vi "Write FPGA Setup Params to File.vi"(8 "error in (no error)":errorcluster, 11 "Path":path) -> (0 "error out":errorcluster)   [LabVIEW 2015, in "Tool Cfg.lvlib"]
uses:
  Tool Cfg.lvlib
  <vilib>/Utility/xml.llb/Write to XML File(array).vi
  Tool Module/Tool Module.lvlib
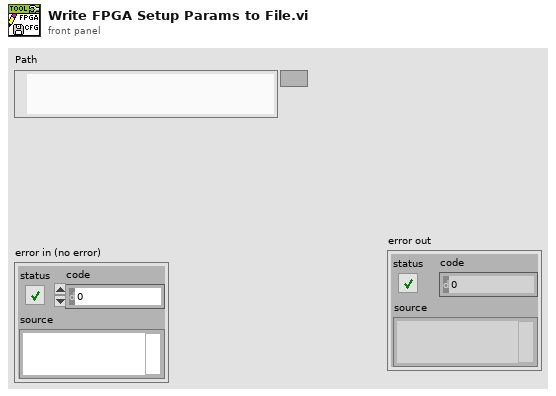
[diagram p1: front panel]
types:
  T1 = typedef "Tool Module.lvlib/Get FPGA Setup Params (Reply Payload)--cluster.ctl" = cluster{"Version String":string, "FPGA Setup Parameters":T2}
  T2 = typedef "_FPGA Setup Params Cluster--typedef.ctl" = cluster{"FPGA Timing Constraints":T3, "FPGA Timing Ctrl":T4, "FPGA Laser Config":T5, "FPGA Peak Proc Cfg":T6, "FPGA SPI Cfg":T7}
  T3 = typedef "_FPGA Timing Constraints Cluster--typedef.ctl" = cluster{"frame.length Min":u16, "frame.ST_OFF Min":u16, "frame.ST_ON Min":u16, "frame.first data idx":u16, "frame.integ Offset":u16, "frame.integ Delay":u16, "frame.ad_latch Delay":u16, "frame.trig time Max":u32}
  T4 = typedef "_FPGA Timing Ctrl Cluster--typedef.ctl" = cluster{"trig.time":u32, "integ.count 1":u32, "integ.count 2":u32, "encdr.latch ctrl":u32, "pixel.read count":u16, "clock.select":u16, "ad.clock offset":u16, "data.control reg":u16}
  T5 = typedef "_FPGA Laser Config Cluster--typedef.ctl" = cluster{"laser.gain":i16, "laser.threshold Low":u16, "laser.threshold High":u16, "laser.dac init":u16, "laser.dac Min":u16, "laser.dac Max":u16, "laser.config reg":u16}
  T6 = typedef "_FPGA Peak Proc Cfg Cluster--typedef.ctl" = cluster{"PD.threshold":u16, "PD.width detect Min":u8, "PD.sensor pixels":u16, "PD.config reg":u16}
  T7 = typedef "_FPGA SPI Cfg Cluster--typedef.ctl" = cluster{"SPI Divide Value":u8, "SPI config reg":u16}
  T8 = typedef "Tool Module.lvlib/Get Mtrl Ctrl Reg (Reply Payload)--cluster.ctl" = cluster{"Mtr Ctrl Reg":u16, "Get Mtrl Ctrl Reg_error":errorcluster}
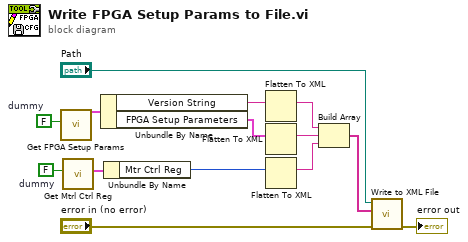
[diagram p0: block diagram]
diagram:
  w2 = FALSE  # dummy
  w5 = FALSE  # dummy
  n1 = call "Get FPGA Setup Params.vi"("dummy"=w5) -> ("Reply Payload"=w14:T1)  [unwired: 8 in, 2 out]
  n2 = call "Get Mtrl Ctrl Reg.vi"("dummy"=w2) -> ("Reply Payload"=w4:T8)  [unwired: 8 in, 2 out]
  n3 = Unbundle By Name(w14) -> ("Version String"=w13:string, "FPGA Setup Parameters"=w12:T2)
  n4 = Unbundle By Name(w4) -> ("Mtr Ctrl Reg"=w3:u16)
  n5 = Flatten To XML(anything=w13) -> (xml string=w11:string)
  n6 = Flatten To XML(anything=w12) -> (xml string=w10:string)
  n7 = Flatten To XML(anything=w3) -> (xml string=w1:string)
  n8 = Build Array(w11, w10, w1) -> (w9:string[])
  n9 = call-poly <vilib>:"Write to XML File.vi"("error in (no error)"="error in (no error)", "XML Input"=w9, "XML File Path"="Path") -> ("error out"=→"error out":errorcluster)  [unwired: 6 in, 2 out]
